vi "Clusters.vi"() -> ()   [LabVIEW 2012]
panel:
  out "output cluster":T1
  in  "Numeric":dbl
  out "Student Data":T2
  in  "Male/Female":cluster{"Boolean":bool}
  in  "Name":cluster{"String":string}
  in  "Roll Number":cluster{"Numeric":dbl}
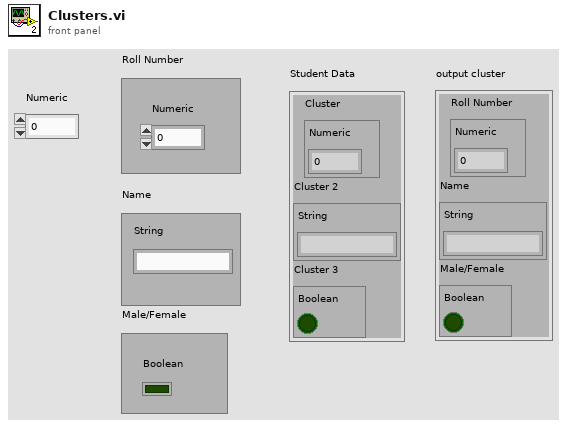
[diagram p1: front panel]
types:
  T1 = cluster{"Roll Number":cluster{"Numeric":dbl}, "Name":cluster{"String":string}, "Male/Female":cluster{"Boolean":bool}}
  T2 = cluster{"Cluster":cluster{"Numeric":dbl}, "Cluster 2":cluster{"String":string}, "Cluster 3":cluster{"Boolean":bool}}
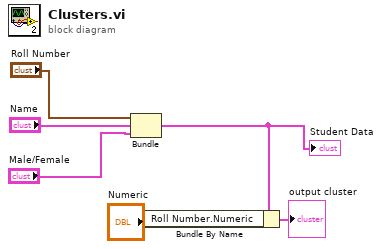
[diagram p0: block diagram]
diagram:
  n1 = Bundle("Roll Number"="Roll Number", "Name"="Name", "Male/Female"="Male/Female") -> (w2:T1)  [unwired: 1 in]
  "Student Data" <- w2
  n2 = Bundle By Name(cluster=w2, "Roll Number.Numeric"="Numeric") -> (→"output cluster":T1)
